vi "期末.vi"() -> ()   [LabVIEW 2014]
uses:
  <vilib>/Utility/inputDevices.llb/keyboardAcquire.vi
  <vilib>/vision/NI_Vision_Development_Module.lvlib
panel:
  in  "停止":bool
  in  "紀錄":bool
  out "subarray":dbl[](array[numeric])
  out "output cluster":cluster{"X":dbl, "Y":dbl}
  out "Number of Particles":i32
  in  "顏色範圍初始化":bool
  in  "1. 範圍選擇":T1={"色相（H）"={0, 255}, "飽和度（S）"={0, 255}, "亮度（L）"={0, 255}} {"亮度（L）" scale=0.0..255.0; "飽和度（S）" scale=0.0..255.0; "色相（H）" scale=0.0..255.0}
  in  "Tab Control":T2(tab)
  out "1. 顏色選取":T3(plugin-control)
  out "2. 填補空隙":T3(plugin-control)
  out "3. 移除雜點":T3(plugin-control)
  out "4. 形狀修正":T3(plugin-control)
  out "5. 選取結果":T3(plugin-control)
  out "Particle Measurements":dbl[][](array[numeric])
  out "Error Out":errorcluster
  in  "3. Number of Erosion":i32=10
  out "滑鼠位置顏色":T4
  in  "Stop Button":bool
  out "0. 原始畫面":T3(plugin-control)
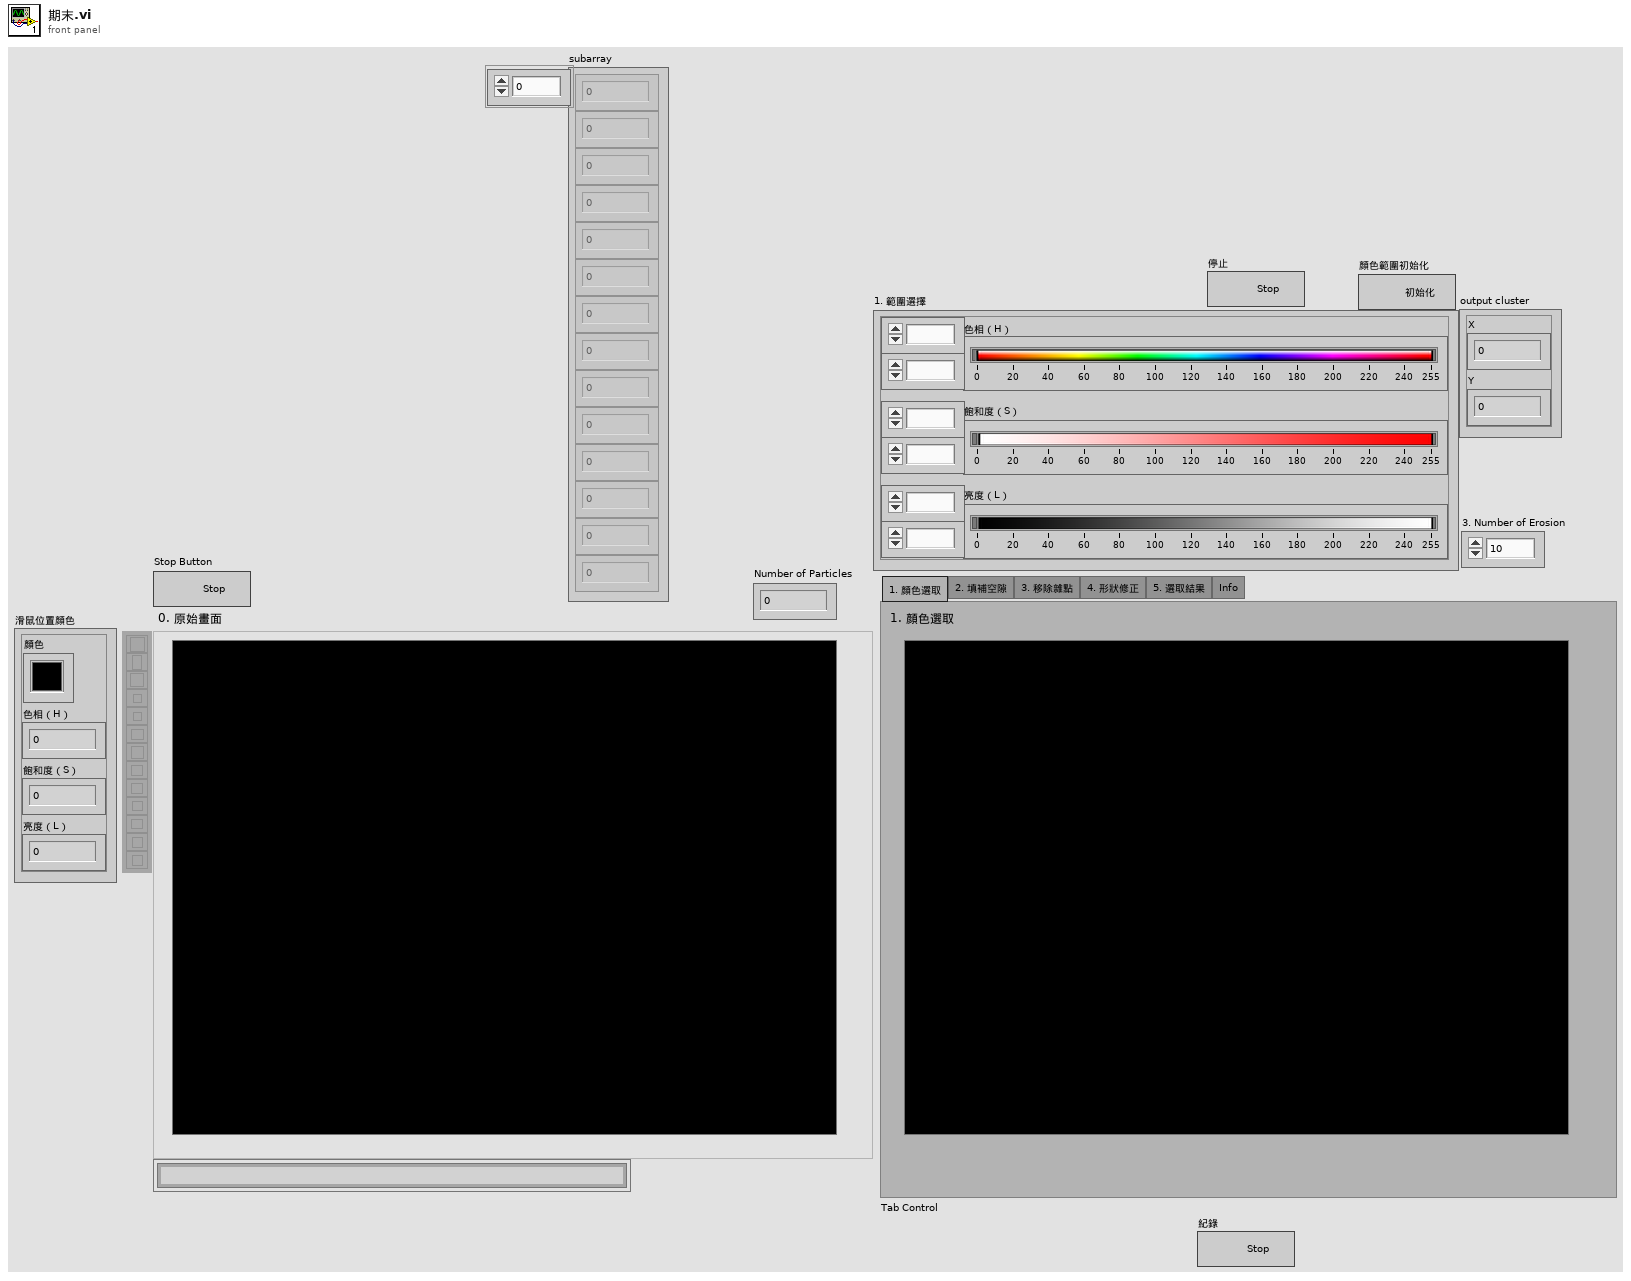
[diagram p1: front panel]
types:
  T1 = cluster{"色相（H）":cluster{u8, u8}, "飽和度（S）":cluster{u8, u8}, "亮度（L）":cluster{u8, u8}}
  T2 = enum32{"1. 顏色選取", "2. 填補空隙", "3. 移除雜點", "4. 形狀修正", "5. 選取結果", "Info"}
  T3 = typedef "IMAQ Image.ctl" = refnum<image>
  T4 = cluster{"色相（H）":u8, "飽和度（S）":u8, "亮度（L）":u8, "顏色":u32}
  T5 = enum16{"0", "1", "2", "3", "4", "5", "6", "7", "8", "9", "A", "B", "C", "D", "E", "F", "G", "H", "I", "J", "K", "L", "M", "N", "O", "P", "Q", "R", "S", "T", "U", "V", "W", "X", "Y", "Z", "F1", "F2", "F3", "F4", "F5", "F6", "F7", "F8", "F9", "F10", "F11", "F12", "F13", "F14", "F15", "ADD", "BACK", "BACKSLASH", "CAPITAL", "COMMA", "DECIMAL", "DELETE", "DIVIDE", "DOWN", "END", "EQUALS", "ESCAPE", "GRAVE (`)", "HOME", "INSERT", "LBRACKET", "LCONTROL", "LEFT", "L ALT", "LSHIFT", "LWIN", "MINUS", "MULTIPLY", "NEXT", "NUMLOCK", "NUMPAD_0", "NUMPAD_1", "NUMPAD_2", "NUMPAD_3", "NUMPAD_4", "NUMPAD_5", "NUMPAD_6", "NUMPAD_7", "NUMPAD_8", "NUMPAD_9", "PAUSE", "PERIOD", "PRIOR (PG UP)", "RBRACKET", "RCONTROL", "RETURN", "RIGHT", "R ALT", "RSHIFT", "RWIN", "SCROLL", "SEMICOLON", "SLASH", "SPACE", "SUBTRACT", "TAB", "UP", "ENTER (num pad)", "' (quote)"}[]
  T6 = enum16{"0", "1", "2", "3", "4", "5", "6", "7", "8", "9", "A", "B", "C", "D", "E", "F", "G", "H", "I", "J", "K", "L", "M", "N", "O", "P", "Q", "R", "S", "T", "U", "V", "W", "X", "Y", "Z", "F1", "F2", "F3", "F4", "F5", "F6", "F7", "F8", "F9", "F10", "F11", "F12", "F13", "F14", "F15", "ADD", "BACK", "BACKSLASH", "CAPITAL", "COMMA", "DECIMAL", "DELETE", "DIVIDE", "DOWN", "END", "EQUALS", "ESCAPE", "GRAVE (`)", "HOME", "INSERT", "LBRACKET", "LCONTROL", "LEFT", "L ALT", "LSHIFT", "LWIN", "MINUS", "MULTIPLY", "NEXT", "NUMLOCK", "NUMPAD_0", "NUMPAD_1", "NUMPAD_2", "NUMPAD_3", "NUMPAD_4", "NUMPAD_5", "NUMPAD_6", "NUMPAD_7", "NUMPAD_8", "NUMPAD_9", "PAUSE", "PERIOD", "PRIOR (PG UP)", "RBRACKET", "RCONTROL", "RETURN", "RIGHT", "R ALT", "RSHIFT", "RWIN", "SCROLL", "SEMICOLON", "SLASH", "SPACE", "SUBTRACT", "TAB", "UP", "ENTER (num pad)", "' (quote)"}
  T7 = cluster{"Numeric":dbl, "Numeric":dbl, "Numeric":dbl, "Numeric":dbl}
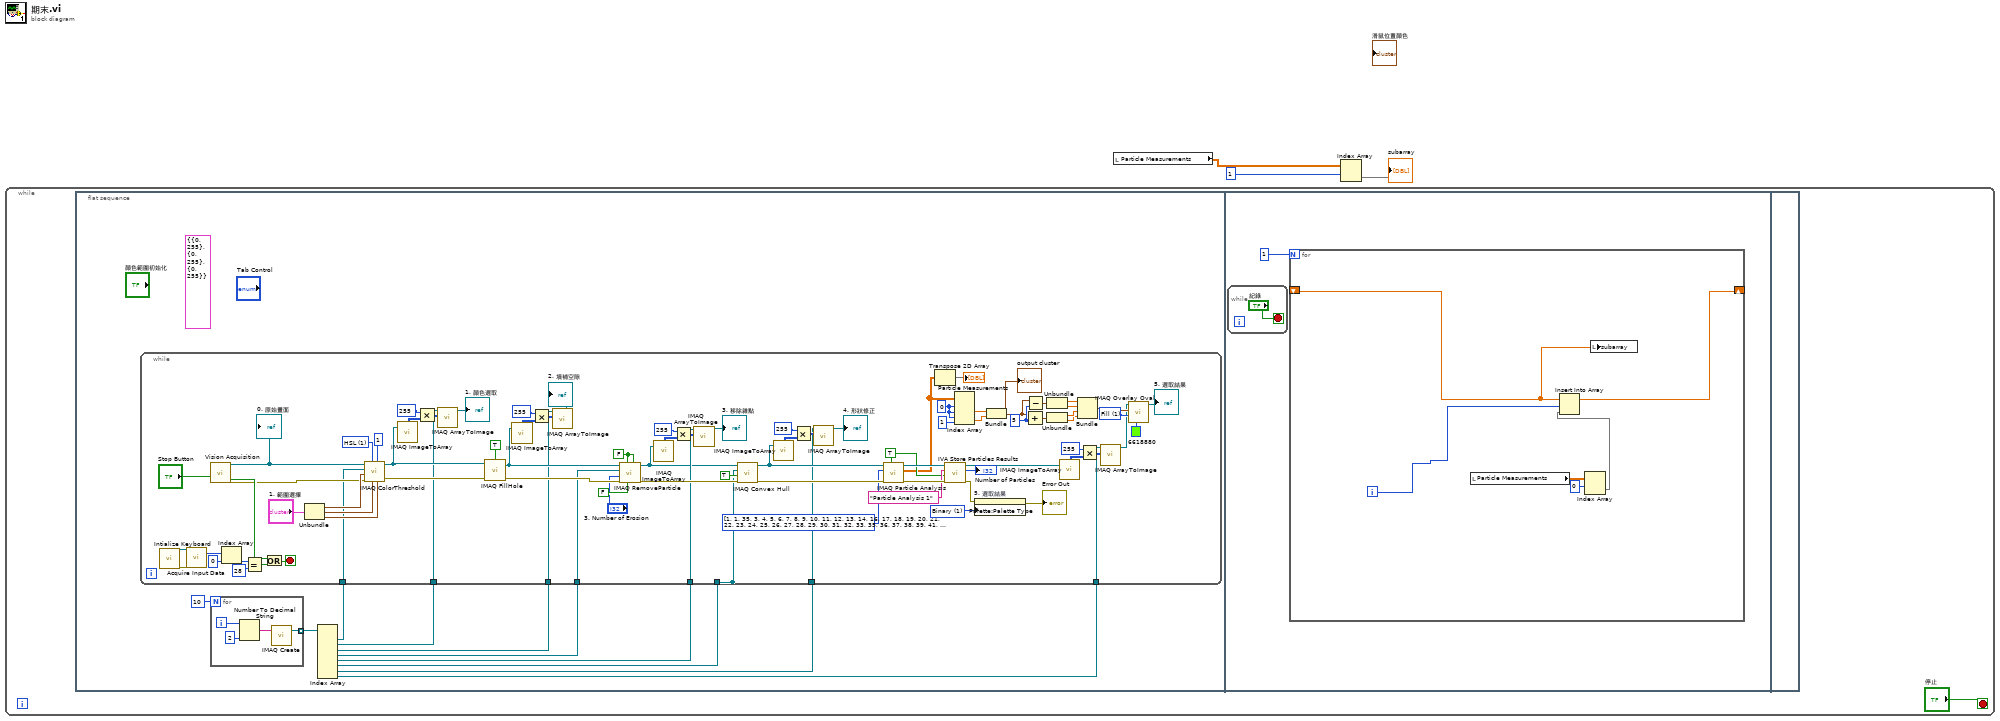
[diagram p0: block diagram]
diagram:
  n1 = while {
    stop <- "停止" stop-if-true
    n2 = flat-sequence {
      frame #0 {
        (unwired) T1 {"色相（H）"={0, 255}, "飽和度（S）"={0, 255}, "亮度（L）"={0, 255}} ("範圍選擇")
        n3 = for {
          N: 10 -> [_]
          tunnel: [w15] -> w14 mode=indexing
          i -> [w17]
          n4 = Number To Decimal String(number=w17, width (-)=2) -> (decimal integer string=w16:string)
          n5 = call "IMAQ Create"("Image Name"=w16) -> ("New Image"=w15:T3)  [unwired: 4 in, 1 out]
        }
        n6 = Index Array(array=w14) -> (element #1=w13:T3, element #2=w12:T3, element #3=w11:T3, element #4=w9:T3, element #5=w8:T3, element #6=w7:T3, element #7=w6:T3, element #8=w5:T3)  [unwired: 8 in]
        n7 = while {
          tunnel: w11 -> [w57]
          tunnel: w9 -> [w72]
          tunnel: w7 -> [w70]
          tunnel: [w70] -> _
          tunnel: w12 -> [w64]
          tunnel: w13 -> [w56]
          tunnel: w8 -> [w52]
          tunnel: w6 -> [w44]
          tunnel: w5 -> [w21]
          stop <- w96 stop-if-true
          w26 = u32 1 items=["Frame", "Fill"] ("Drawing Mode (Frame)")
          w35 = 5
          w40 = 0
          w73 = u32 1 items=["Grayscale", "Binary", "Gradient", "Rainbow", "Temperature", "User Defined"] ("Palette")
          w82 = i32[] [1, 1, 35, 3, 4, 5, 6, 7, 8, 9, 10, 11, 12, 13, 14, 16, 17, 18, 19, 20, 21, 22, 23, 24, 25, 26, 27, 28, 29, 30, 31, 32, 33, 35, 36, 37, 38, 39, 41, 42, 43, 45, 46, 48, 49, 50, 51, 53, 54, 55, 56, 58, 59, 60, 61, 62, 63, 64, 65, 66, 68, 69, 70, 71, 72, 73, 74, 75, 76, 77, 78, 79, 80, 81, 82, 83, 84, 85, 86, 87, 88] items=["Center of Mass X", "Center of Mass Y", "First Pixel X", "First Pixel Y", "Bounding Rect Left", "Bounding Rect Top", "Bounding Rect Right", "Bounding Rect Bottom", "Max Feret Diameter Start X", "Max Feret Diameter Start Y", "Max Feret Diameter End X", "Max Feret Diameter End Y", "Max Horiz. Segment Length Left", "Max Horiz. Segment Length Right", "Max Horiz. Segment Length Row", "-", "Bounding Rect Width", "Bounding Rect Height", "Bounding Rect Diagonal", "Perimeter", "Convex Hull Perimeter", "Holes' Perimeter", "Max Feret Diameter", "Equivalent Ellipse Major Axis", "Equivalent Ellipse Minor Axis", "Equivalent Ellipse Minor Axis (Feret)", "Equivalent Rect Long Side", "Equivalent Rect Short Side", "Equivalent Rect Diagonal", "Equivalent Rect Short Side (Feret)", "Average Horiz. Segment Length", "Average Vert. Segment Length", "Hydraulic Radius", "Waddel Disk Diameter", "-", "Area", "Holes' Area", "Particle & Holes' Area", "Convex Hull Area", "Image Area", "-", "Number of Holes", "Number of Horiz. Segments", "Number of Vert. Segments", "-", "Orientation", "Max Feret Diameter Orientation", "-", "% Area/Image Area", "% Area/(Particle & Holes' Area)", "Ratio of Equivalent Ellipse Axes", "Ratio of Equivalent Rect Sides", "-", "Elongation Factor", "Compactness Factor", "Heywood Circularity Factor", "Type Factor", "-", "Sum X", "Sum Y", "Sum XX", "Sum XY", "Sum YY", "Sum XXX", "Sum XXY", "Sum XYY", "Sum YYY", "-", "Moment of Inertia XX", "Moment of Inertia XY", "Moment of Inertia YY", "Moment of Inertia XXX", "Moment of Inertia XXY", "Moment of Inertia XYY", "Moment of Inertia YYY", "Norm. Moment of Inertia XX", "Norm. Moment of Inertia XY", "Norm. Moment of Inertia YY", "Norm. Moment of Inertia XXX", "Norm. Moment of Inertia XXY", "Norm. Moment of Inertia XYY", "Norm. Moment of Inertia YYY", "Hu Moment 1", "Hu Moment 2", "Hu Moment 3", "Hu Moment 4", "Hu Moment 5", "Hu Moment 6", "Hu Moment 7"] ("Pixel Measurements")
          w84 = TRUE ("Connectivity 4/8 (8)")
          w63 = FALSE ("Connectivity 4/8 (8)")
          w93 = u16 1 items=["RGB", "HSL", "HSV", "HSI"] ("Color Mode")
          n8 = call <vilib>:"Intialize Keyboard.vi"() -> ("error out"=w100:errorcluster, "device ID"=w101:refnum<k1>)  [unwired: 10 in]
          n9 = call-poly <vilib>:"Acquire Input Data.vi"("device ID"=w101, "error in (no error)"=w100) -> ("keys pressed"=w102:T5)  [unwired: 15 in, 2 out]
          n10 = call "Vision Acquisition"("Stop (F)"="Stop Button") -> ("Image Out"=w95:T3, "Stopped"=w97:bool, "error out"=w88:errorcluster)  [unwired: 24 in]
          "0. 原始畫面" <- w95
          n11 = Index Array(array=w102, index=0) -> (element=w105:T6)
          n12 = Equal?(x=w105, y=28) -> (x = y?=w99:bool)
          n13 = Or(x=w97, y=w99) -> (x .or. y?=w96:bool)
          n14 = Unbundle("1. 範圍選擇") -> ("色相（H）"=w92:cluster{u8, u8}, "飽和度（S）"=w91:cluster{u8, u8}, "亮度（L）"=w90:cluster{u8, u8})
          n15 = call "IMAQ ColorThreshold"("Blue or Luma or Val or Inten Range"=w90, "Replace Value"=1, "Green or Sat Range"=w91, "Color Mode"=w93, "error in (no error)"=w88, "Red or Hue Range"=w92, "Image Dst"=w56, "Image Src"=w95) -> ("error out"=w75:errorcluster, "Image Dst Out"=w69:T3)  [unwired: 2 out]
          n16 = call "IMAQ ImageToArray"("Image"=w69) -> ("Image Pixels (U8)"=w67:u8[][])  [unwired: 3 in, 4 out]
          n17 = Multiply(x=255, y=w67) -> (x*y=w66:i32[][])
          n18 = call "IMAQ ArrayToImage"("Image Pixels (U8)"=w66, "Image"=w64) -> ("Image Out"=→"1. 顏色選取":T3)  [unwired: 8 in, 1 out]
          n19 = call "IMAQ FillHole"("error in (no error)"=w75, "Image Src"=w69, "Connectivity 4/8 (8)"=TRUE) -> ("error out"=w79:errorcluster, "Image Dst Out"=w58:T3)  [unwired: 1 in, 2 out]
          n20 = call "IMAQ ImageToArray"("Image"=w58) -> ("Image Pixels (U8)"=w61:u8[][])  [unwired: 3 in, 4 out]
          n21 = Multiply(x=255, y=w61) -> (x*y=w62:i32[][])
          n22 = call "IMAQ ArrayToImage"("Image Pixels (U8)"=w62, "Image"=w57) -> ("Image Out"=→"2. 填補空隙":T3)  [unwired: 8 in, 1 out]
          n23 = call "IMAQ RemoveParticle"("Connectivity 4/8 (8)"=w63, "Low Pass/High Pass (Low)"=FALSE, "Square/Hexa (Square)"=w63, "error in (no error)"=w79, "Number of Erosion"="3. Number of Erosion", "Image Dst"=w72, "Image Src"=w58) -> ("error out"=w80:errorcluster, "Image Dst Out"=w50:T3)  [unwired: 3 out]
          n24 = call "IMAQ ImageToArray"("Image"=w50) -> ("Image Pixels (U8)"=w54:u8[][])  [unwired: 3 in, 4 out]
          n25 = Multiply(x=255, y=w54) -> (x*y=w53:i32[][])
          n26 = call "IMAQ ArrayToImage"("Image Pixels (U8)"=w53, "Image"=w52) -> ("Image Out"=→"3. 移除雜點":T3)  [unwired: 8 in, 1 out]
          n27 = call "IMAQ Convex Hull"("error in (no error)"=w80, "Connectivity 4/8 (8)"=TRUE, "Image Dst"=w70, "Image Src"=w50) -> ("error out"=w83:errorcluster, "Image Dst Out"=w45:T3)  [unwired: 6 out]
          n28 = call "IMAQ ImageToArray"("Image"=w45) -> ("Image Pixels (U8)"=w48:u8[][])  [unwired: 3 in, 4 out]
          n29 = Multiply(x=255, y=w48) -> (x*y=w49:i32[][])
          n30 = call "IMAQ ArrayToImage"("Image Pixels (U8)"=w49, "Image"=w44) -> ("Image Out"=→"4. 形狀修正":T3)  [unwired: 8 in, 1 out]
          n31 = call "IMAQ Particle Analysis"("Connectivity 4/8 (8)"=w84, "error in (no error)"=w83, "Pixel Measurements"=w82, "Image"=w45) -> ("error out"=w87:errorcluster, "Particle Measurements (Pixels)"=w41:dbl[][], "Image Out (duplicate)"=w85:T3)  [unwired: 1 in, 4 out]
          n32 = Transpose 2D Array(2D array=w41) -> (transposed array=→"Particle Measurements":dbl[][])
          n33 = call <vilib>:"IVA Store Particles Results.vi"("error in (no error)"=w87, "Connectivity 4/8 (8)"=w84, "Step Name"="Particle Analysis 1", "Image in"=w85) -> ("error out"=w74:errorcluster, "Number of Particles"=→"Number of Particles":i32, "Image dup"=w25:T3)  [unwired: 5 out]
          n34 = Index Array(array=w41, index (row) #1=w40, index (col) #1=w40, index (row) #2=w40, index (col) #2=1) -> (element #1=w38:dbl, element #2=w37:dbl)
          n35 = property on="5. 選取結果" class="ImageControl"(error in=w74, "Palette:Palette Type"=w73) -> (error out=→"Error Out":errorcluster)  [unwired: 1 in, 1 out]
          n36 = Bundle("Numeric"=w38, "Numeric"=w37) -> (w34:cluster{"Numeric":dbl, "Numeric":dbl})  [unwired: 1 in]
          "output cluster" <- w34
          n37 = Add(x=w34, y=w35) -> (x+y=w32:cluster{"Numeric":dbl, "Numeric":dbl})
          n38 = Subtract(x=w34, y=w35) -> (x-y=w33:cluster{"Numeric":dbl, "Numeric":dbl})
          n39 = Unbundle(w33) -> ("Numeric"=w31:dbl, "Numeric"=w30:dbl)
          n40 = Unbundle(w32) -> ("Numeric"=w29:dbl, "Numeric"=w28:dbl)
          n41 = call "IMAQ ImageToArray"("Image"=w25) -> ("Image Pixels (U8)"=w22:u8[][])  [unwired: 3 in, 4 out]
          n42 = Bundle("Numeric"=w31, "Numeric"=w30, "Numeric"=w29, "Numeric"=w28) -> (w27:T7)  [unwired: 1 in]
          n43 = Multiply(x=255, y=w22) -> (x*y=w23:i32[][])
          n44 = call "IMAQ ArrayToImage"("Image Pixels (U8)"=w23, "Image"=w21) -> ("Image Out"=w20:T3)  [unwired: 8 in, 1 out]
          n45 = call "IMAQ Overlay Oval"("Color"=u32 6618880, "Drawing Mode (Frame)"=w26, "Bounding Rectangle"=w27, "Image"=w20) -> ("Image Out"=→"5. 選取結果":T3)  [unwired: 6 in, 1 out]
        }
      }
      frame #1 {
        n46 = while {
          stop <- "紀錄" stop-if-true
        }
        n47 = for {
          N: 1 -> [_]
          shift-right: [w113] -> _
          shift-left: _ -> [w109]
          i -> [w108]
          n48 = local read "Particle Measurements"() -> (w112:dbl[][])
          n49 = Index Array(array=w112, index (row)=0) -> (element=w110:dbl[])  [unwired: 1 in]
          n50 = Insert Into Array(array=w109, index=w108, new element=w110) -> (w113:dbl[])
          n51 = local write "subarray"(w109) -> ()
        }
      }
      frame #2 {
      }
    }
  }
  n52 = local read "Particle Measurements"() -> (w1:dbl[][])
  n53 = Index Array(array=w1, index (row)=1) -> (element=→"subarray":dbl[])  [unwired: 1 in]
